vi "Launch.vi"(8 "error in (no error)":errorcluster, 10 "Enqueuer ID string in":string, 11 "Sequencer Core in":refnum<class "Sequencer Core.lvclass">) -> (0 "error out":errorcluster, 3 "Sequencer Core out":refnum<class "Sequencer Core.lvclass">)   [LabVIEW 2020, in "Sequencer.lvlib" / "Sequencer Core.lvclass"]
doc: "Initialize the 'Message Priority Queue, the Interrupt Notifier and then calls Cores 'Pre Launch Init'."
uses:
  Sequencer Core.lvclass
  Sequencer Core.lvclass/Sequencer Core.ctl
  Message Priority Queue/Message Priority Queue.lvclass
  PPL/HDH.Data.Generic.lvlibp/Synchronization/Notifier/Notifier.lvclass
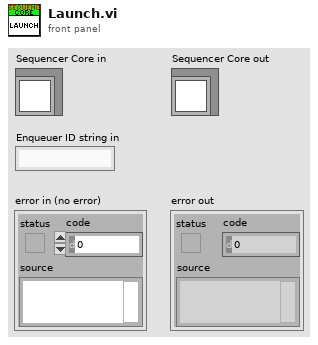
[diagram p1: front panel]
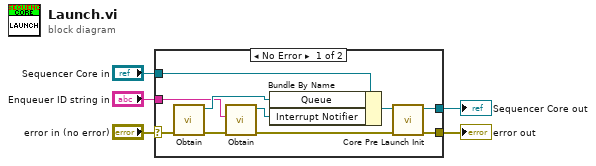
[diagram p0: block diagram]
diagram:
  n1 = case shown="No Error" "error in (no error)" {
    selector: "error in (no error)" -> [w13 w17]
    tunnel: [w7 w17] -> w4
    tunnel: [w9 w16] -> w2
    tunnel: "Sequencer Core in" -> [w15 w16]
    tunnel: "Enqueuer ID string in" -> [w6 _]
    frame No Error {
      n2 = call "Obtain.vi"("error in (no error)"=w13) -> ("error out"=w11:errorcluster, "Priority Queue"=w14:refnum<class "Message Priority Queue.lvclass">)  [unwired: 9 in]
      n3 = call "Obtain.vi"("error in (no error)"=w11, "Name (\"\")"=w6) -> ("error out"=w8:errorcluster, "Notifier out"=w12:refnum<class "Notifier.lvclass">)  [unwired: 7 in, 1 out]
      n4 = Bundle By Name(cluster=w15, "Queue"=w14, "Interrupt Notifier"=w12) -> (w10:refnum<class "Sequencer Core.lvclass">)
      n5 = call-dynamic "Core Pre Launch Init.vi"("error in (no error)"=w8, "Sequencer Core in"=w10) -> ("error out"=w7:errorcluster, "Sequencer Core out"=w9:refnum<class "Sequencer Core.lvclass">)  [unwired: 8 in]
    }
    frame Error {
    }
  }
  "error out" <- w4
  "Sequencer Core out" <- w2
